vi "Tell.vi"(4 "Priority":bool, 10 "Msg":refnum<class "Msg.lvclass">, 11 "Event Transport in":refnum<class "Event Transport.lvclass">) -> (0 "Error out":errorcluster)   [LabVIEW 2025, in "jettl.lvlib" / "Transport.lvlib" / "Event.lvlib" / "Event Transport.lvclass"]
uses:
  Event Transport.lvclass
  Msg/Msg.lvclass
  Event Transport.lvclass/Event Transport.ctl
  <vilib>/event_ctls.llb/usereventprio.ctl
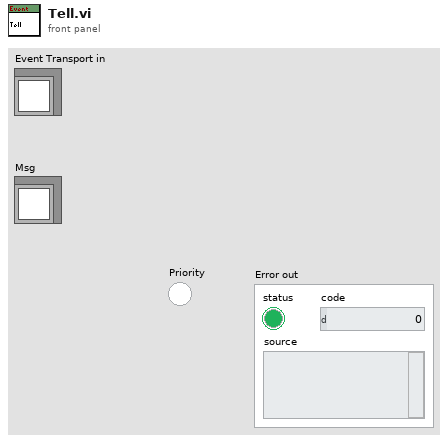
[diagram p1: front panel]
types:
  T1 = typedef "usereventprio.ctl" = enum32{"high priority", "normal priority"}
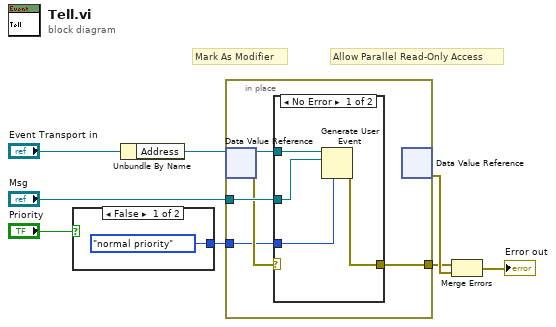
[diagram p0: block diagram]
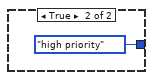
[diagram p3: hidden frame]
diagram:
  # "Allow Parallel Read-Only Access"
  # "Mark As Modifier"
  n1 = case shown="False" "Priority" {
    tunnel: [usereventprio."normal priority" ("priority (normal)") usereventprio."high priority" ("priority (normal)")] -> w3
    frame False {
    }
    frame True {
    }
  }
  n2 = Unbundle By Name("Event Transport in") -> ("Address"=w4:refnum<data-value>)
  n3 = in-place {
    in-place-border: [w15] -> w5
    in-place-border: "Msg" -> [w14]
    in-place-border: w3 -> [w11]
    n4 = in-place-dvr #1(w4) -> (w13:refnum<user-event>, w12:errorcluster)
    n5 = case shown="No Error" w12 {
      selector: w12 -> [_ w20]
      tunnel: [w17 w20] -> w15
      tunnel: w14 -> [w18 _]
      tunnel: w13 -> [w19 _]
      tunnel: w11 -> [w16 _]
      frame No Error {
        n6 = Generate User Event(priority (normal)=w16, user event=w19, event data cluster=w18) -> (error out=w17:errorcluster)  [unwired: 1 in, 1 out]
      }
      frame Error {
      }
    }
    n7 = in-place-dvr #1() -> (w6:errorcluster)  [unwired: 1 in, 1 out]
  }
  n8 = Merge Errors(w5, w6) -> (→"Error out":errorcluster)
